vi "Begin.vi"(8 "error in":errorcluster) -> (0 "error out":errorcluster)   [LabVIEW 2014]
doc: "Called before other user functions, this VI is expected to open initial I/O refnums, load in file data, and do all program initialization. Notice that the <B>error out</B> terminal is simply used for data flow. Wiring it to other structures or subVIs ensures that this VI runs first."
uses:
  <vilib>/Rock Robotics/WPI/DriverStation/WPI_DriverStationRobotMode2.ctl
  <vilib>/Rock Robotics/WPI/Joystick/WPI_JoystickDeviceEnum.ctl
  <vilib>/Rock Robotics/SystemInterfaces/DIO/FPGA_DIOChannel.ctl
  <vilib>/Rock Robotics/SystemInterfaces/Typedef/FPGA_TypedefDigitalModule.ctl
  <vilib>/Rock Robotics/WPI/SafetyOutput/WPI_SafetyOutputConfigMenu.ctl
  <vilib>/Rock Robotics/SystemInterfaces/DIO/FPGA_DIOPWMChannel.ctl
  <vilib>/Rock Robotics/WPI/Solenoid/WPI_SolenoidChannel.ctl
  Robot Global Data.vi
  <vilib>/Rock Robotics/Network Tables/SD Write String Array.vi
  <vilib>/Rock Robotics/WPI/RobotDrive/WPI_RobotDriveOpen4MotorWithCANTalonSRX.vi
  <vilib>/Rock Robotics/WPI/RobotDrive/WPI_RobotDriveOpen2MotorWithCANTalonSRX.vi
  <vilib>/Rock Robotics/WPI/Switch/WPI_SwitchOpenLimit.vi
  <vilib>/Rock Robotics/WPI/Solenoid/WPI_SolenoidOpenDouble.vi
  <vilib>/Rock Robotics/WPI/Compressor/WPI_CompressorGetSetRefNum.vi
  <vilib>/Rock Robotics/WPI/MotorControl/WPI_MotorControlOpen VictorSP.vi
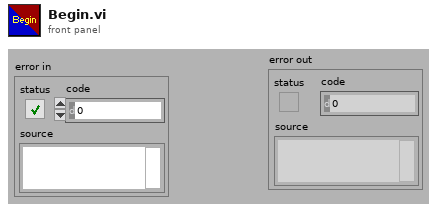
[diagram p1: front panel]
types:
  T1 = typedef "WPI_SolenoidChannel.ctl" = enum8{"Solenoid 0", "Solenoid 1", "Solenoid 2", "Solenoid 3", "Solenoid 4", "Solenoid 5", "Solenoid 6", "Solenoid 7", "Invalid"}
  T2 = typedef "FPGA_DIOChannel.ctl" = enum8{"DIO 0", "DIO 1", "DIO 2", "DIO 3", "DIO 4", "DIO 5", "DIO 6", "DIO 7", "DIO 8", "DIO 9", "DIO MXP 0", "DIO MXP 1", "DIO MXP 2", "DIO MXP 3", "DIO MXP 4", "DIO MXP 5", "DIO MXP 6", "DIO MXP 7", "DIO MXP 8", "DIO MXP 9", "DIO MXP 10", "DIO MXP 11", "DIO MXP 12", "DIO MXP 13", "DIO MXP 14", "DIO MXP 15", "Invalid"}
  T3 = typedef "FPGA_TypedefDigitalModule.ctl" = enum16{"Controller 1"}
  T4 = typedef "FPGA_DIOPWMChannel.ctl" = enum8{"PWM 0", "PWM 1", "PWM 2", "PWM 3", "PWM 4", "PWM 5", "PWM 6", "PWM 7", "PWM 8", "PWM 9", "PWM MXP 0", "PWM MXP 1", "PWM MXP 2", "PWM MXP 3", "PWM MXP 4", "PWM MXP 5", "PWM MXP 6", "PWM MXP 7", "PWM MXP 8", "PWM MXP 9", "Invalid"}
  T5 = typedef "WPI_SafetyOutputConfigMenu.ctl" = enum16{"Enable", "Disable"}
  T6 = typedef "WPI_JoystickDeviceEnum.ctl" = enum16{"USB 0", "USB 1", "USB 2", "USB 3", "USB 4", "USB 5"}
  T7 = typedef "WPI_DriverStationRobotMode2.ctl" = enum16{"Autonomous Disabled", "Autonomous Enabled", "Teleop Disabled", "Teleop Enabled", "Disconnected", "Finish", "Test Disabled", "Test Enabled", "Emergency Stopped"}
  T8 = typedef "WPI_MotorControlDeviceRef.ctl" = cluster{"DeviceStatus":errorcluster, "Type":T9, "PWM":cluster{"Controller":T3, "PWM Channel":T4, "DeadBand":T10}, "CAN":cluster{"Device Number":u8, "Control Mode":T11, "Semaphore":T12, "Max Vout":dbl, "TalonSRX Control Mode":T13}, "Invert":bool, "TransformRef":T14, "InvTransformRef":T14}
  T9 = typedef "WPI_MotorControlType.ctl" = enum16{"PWM", "CAN", "CANTalonSRX"}
  T10 = typedef "WPI_PWMDeadband.ctl" = cluster{"Name":string, "maxPositivePwm":i32, "minPositivePwm":i32, "centerPwm":i32, "maxNegativePwm":i32, "minNegativePwm":i32, "angularRange":u16}
  T11 = typedef "WPI_CANJaguar_ControlMode.ctl" = enum8{"Percent VBus", "Current", "Speed", "Position", "Voltage"}
  T12 = typedef "Semaphore RefNum" = refnum<k1>
  T13 = typedef "WPI_CANTalonSRX_APIControlMode.ctl" = enum8{"Percent VBus", "Speed", "Position", "Slave", "Unchanged / Invalid"}
  T14 = typedef "WPI_PWMTransform_ConPane.ctl" = refnum<vi>
  T15 = typedef "WPI_RobotDriveDevRef.ctl" = cluster{"DevStatus":errorcluster, "Motors[]":T8[], "Square Inputs":bool, "Max Output":dbl}
  T16 = typedef "WPI_CompressorDevRef.ctl" = cluster{"DevStatus":errorcluster, "Pneumatics Control Module":u8}
  T17 = typedef "WPI_ServoDeviceRef.ctl" = cluster{"DeviceStatus":errorcluster, "Controller":T3, "PWM Channel":T4, "DeadBand":T10}
  T18 = typedef "WPI_JoystickDevRef.ctl" = cluster{"Device":T6}
  T19 = typedef "WPI_DigitalInputDevRef.ctl" = cluster{"DevStatus":errorcluster, "DIO Channel":T2, "Controller":T3}
  T20 = typedef "WPI_SolenoidDevRef.ctl" = cluster{"DevStatus":errorcluster, "Pneumatics Control Module":u8, "Forward Solenoid Channel":T1, "Reverse Solenoid Channel":T1}
  T21 = typedef "WPI_SwitchDevRef.ctl" = cluster{"DevStatus":errorcluster, "DIO Channel":T2, "Controller":T3, "CntIndex":T22, "Normally Closed":bool}
  T22 = typedef "FPGA_CounterCtrSystemIndex.ctl" = enum8{"Ctr 0", "Ctr 1", "Ctr 2", "Ctr 3", "Ctr 4", "Ctr 5", "Ctr 6", "Ctr 7", "Invalid"}
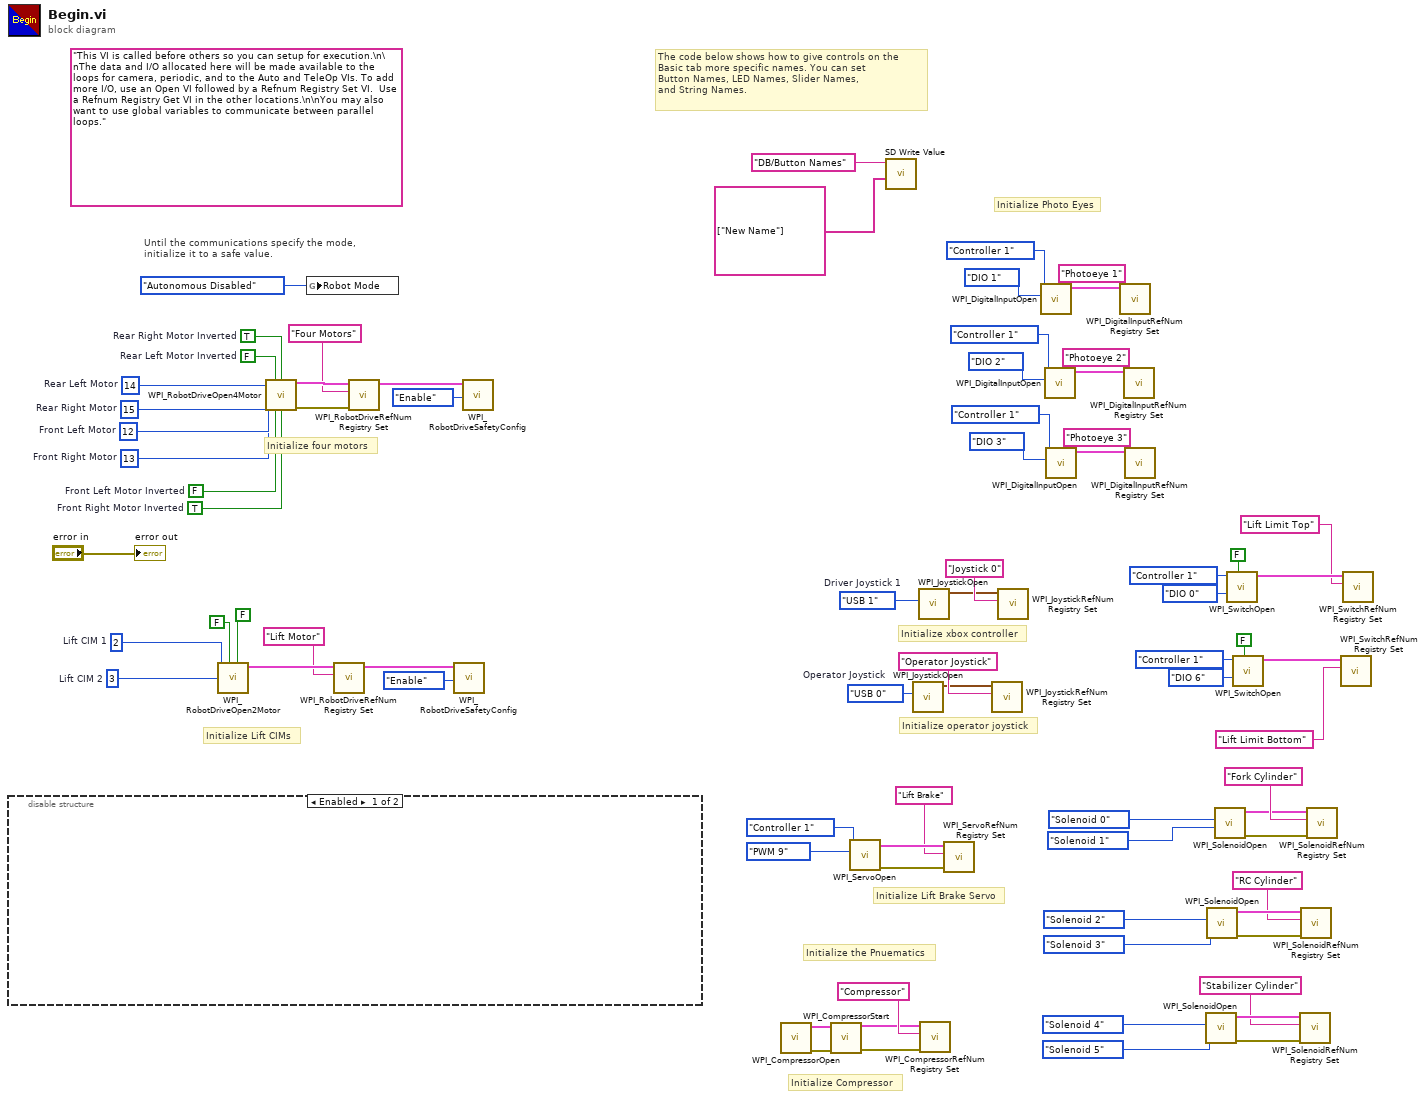
[diagram p0: block diagram]
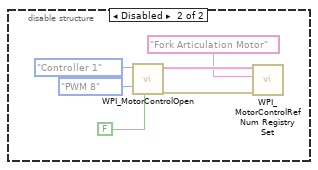
[diagram p2: hidden frame]
diagram:
  w38 = u8 3  # Lift CIM 2
  w37 = u8 2  # Lift CIM 1
  w56 = u8 13  # Front Right Motor
  w57 = u8 12  # Front Left Motor
  w58 = u8 15  # Rear Right Motor
  w59 = u8 14  # Rear Left Motor
  w60 = WPI_JoystickDeviceEnum."USB 0"  # Operator Joystick
  w63 = TRUE  # Front Right Motor Inverted
  w64 = FALSE  # Front Left Motor Inverted
  w65 = TRUE  # Rear Right Motor Inverted
  w66 = FALSE  # Rear Left Motor Inverted
  w70 = WPI_JoystickDeviceEnum."USB 1"  # Driver Joystick 1
  (unwired) "This VI is called before others so you can setup for execution.\n\nThe data and I/O allocated here will be made available to the loops for camera, periodic, and to the Auto and TeleOp VIs. To add more I/O, use an Open VI followed by a Refnum Registry Set VI.  Use a Refnum Registry Get VI in the other locations.\n\nYou may also want to use global variables to communicate between parallel loops."
  # "Initialize Compressor"
  # "Initialize the Pnuematics"
  # "Initialize Photo Eyes"
  # "Initialize Lift Brake Servo"
  # "Initialize Lift CIMs"
  # "Initialize operator joystick"
  # "The code below shows how to give controls on the\nBasic tab more specific names. You can set\nButton Names, LED Names, Slider Names,\nand String Names."
  # "Initialize xbox controller"
  # "Until the communications specify the mode,\ninitialize it to a safe value."
  # "Initialize four motors"
  n1 = disable-structure shown="Enabled" {
    frame Enabled {
    }
    frame Disabled {
      n2 = call-poly <vilib>:"WPI_MotorControlOpen.vi"("Invert"=FALSE, "PWM Channel"=FPGA_DIOPWMChannel."PWM 8", "Controller"=FPGA_TypedefDigitalModule."Controller 1") -> ("error out"=w79:errorcluster, "MotorControlDeviceRef"=w82:T8)  [unwired: 7 in]
      n3 = call <vilib>:"WPI_MotorControlRefNum Registry Set.vi"("error in (no error)"=w79, "refnum name"="Fork Articulation Motor", "MotorControlDevRef"=w82) -> ()  [unwired: 7 in, 2 out]
    }
  }
  n4 = call-poly <vilib>:"WPI_RobotDriveOpen2Motor.vi"("Right Motor Inverted"=FALSE, "Left Motor Inverted"=FALSE, "Right Motor"=w38, "Left Motor"=w37) -> ("RobotDriveDevRef"=w41:T15)  [unwired: 6 in, 1 out]
  n5 = call-poly <vilib>:"WPI_RobotDriveOpen4Motor.vi"("Rear Left Motor"=w59, "Rear Left Motor Inverted"=w66, "Rear Right Motor Inverted"=w65, "Rear Right Motor"=w58, "Front Left Motor"=w57, "Front Right Motor"=w56, "Front Left Motor Inverted"=w64, "Front Right Motor Inverted"=w63) -> ("RobotDriveDevRef"=w78:T15, "error out"=w76:errorcluster)  [unwired: 6 in]
  n6 = global write "Robot Global Data.vi" "Robot Mode"(WPI_DriverStationRobotMode2."Autonomous Disabled" ("Robot Mode")) -> ()
  n7 = call <vilib>:"WPI_RobotDriveRefNum Registry Set.vi"("refnum name"="Lift Motor", "RobotDriveDevRef"=w41) -> ("RobotDriveDevRef"=w43:T15)  [unwired: 8 in, 1 out]
  n8 = call <vilib>:"WPI_RobotDriveRefNum Registry Set.vi"("error in (no error)"=w76, "refnum name"="Four Motors", "RobotDriveDevRef"=w78) -> ("RobotDriveDevRef"=w75:T15)  [unwired: 8 out]
  n9 = call <vilib>:"WPI_RobotDriveSafetyConfig.vi"("mode"=WPI_SafetyOutputConfigMenu."Enable", "RobotDriveDevRef"=w43) -> ()  [unwired: 8 in, 2 out]
  n10 = call <vilib>:"WPI_RobotDriveSafetyConfig.vi"("mode"=WPI_SafetyOutputConfigMenu."Enable", "RobotDriveDevRef"=w75) -> ()  [unwired: 8 in, 2 out]
  n11 = call <vilib>:"WPI_CompressorOpen.vi"() -> ("CompressorDevRef"=w18:T16, "error out"=w11:errorcluster)  [unwired: 14 in]
  n12 = call <vilib>:"WPI_CompressorStart.vi"("error in (no error)"=w11, "CompressorDevRef"=w18) -> ("error out"=w12:errorcluster, "CompressorDevRef"=w13:T16)  [unwired: 8 out]
  n13 = call <vilib>:"WPI_ServoOpen.vi"("PWM Channel"=FPGA_DIOPWMChannel."PWM 9", "Controller"=FPGA_TypedefDigitalModule."Controller 1") -> ("error out"=w21:errorcluster, "ServoDeviceRef"=w33:T17)  [unwired: 8 in]
  n14 = call-poly <vilib>:"SD Write Value.vi"("String Array"=string[] ["New Name"], "Name"="DB/Button Names") -> ()  [unwired: 8 in, 2 out]
  n15 = call <vilib>:"WPI_JoystickOpen.vi"("JoystickDevice"=w60) -> ("JoystickDevRef"=w61:T18)  [unwired: 10 in]
  n16 = call <vilib>:"WPI_JoystickOpen.vi"("JoystickDevice"=w70) -> ("JoystickDevRef"=w71:T18)  [unwired: 10 in]
  n17 = call <vilib>:"WPI_CompressorRefNum Registry Set.vi"("error in (no error)"=w12, "refnum name"="Compressor", "CompressorDevRef"=w13) -> ()  [unwired: 7 in, 2 out]
  n18 = call <vilib>:"WPI_ServoRefNum Registry Set.vi"("error in (no error)"=w21, "refnum name"="Lift Brake", "ServoDeviceRef"=w33) -> ()  [unwired: 7 in, 2 out]
  n19 = call <vilib>:"WPI_JoystickRefNum Registry Set.vi"("refnum name"="Operator Joystick", "JoystickDevRef"=w61) -> ()  [unwired: 8 in, 2 out]
  n20 = call <vilib>:"WPI_JoystickRefNum Registry Set.vi"("refnum name"="Joystick 0", "JoystickDevRef"=w71) -> ()  [unwired: 8 in, 2 out]
  n21 = call <vilib>:"WPI_DigitalInputOpen.vi"("DIO Channel"=FPGA_DIOChannel."DIO 1", "Controller"=FPGA_TypedefDigitalModule."Controller 1") -> ("DigitalInputDevRef"=w47:T19)  [unwired: 8 in, 1 out]
  n22 = call <vilib>:"WPI_DigitalInputOpen.vi"("DIO Channel"=FPGA_DIOChannel."DIO 2", "Controller"=FPGA_TypedefDigitalModule."Controller 1") -> ("DigitalInputDevRef"=w55:T19)  [unwired: 8 in, 1 out]
  n23 = call <vilib>:"WPI_DigitalInputOpen.vi"("DIO Channel"=FPGA_DIOChannel."DIO 3", "Controller"=FPGA_TypedefDigitalModule."Controller 1") -> ("DigitalInputDevRef"=w51:T19)  [unwired: 8 in, 1 out]
  n24 = call <vilib>:"WPI_DigitalInputRefNum Registry Set.vi"("refnum name"="Photoeye 1", "DigitalInputDevRef"=w47) -> ()  [unwired: 8 in, 2 out]
  n25 = call <vilib>:"WPI_DigitalInputRefNum Registry Set.vi"("refnum name"="Photoeye 2", "DigitalInputDevRef"=w55) -> ()  [unwired: 8 in, 2 out]
  n26 = call <vilib>:"WPI_DigitalInputRefNum Registry Set.vi"("refnum name"="Photoeye 3", "DigitalInputDevRef"=w51) -> ()  [unwired: 8 in, 2 out]
  n27 = call-poly <vilib>:"WPI_SolenoidOpen.vi"("Reverse Solenoid Channel"=WPI_SolenoidChannel."Solenoid 5", "Forward Solenoid Channel"=WPI_SolenoidChannel."Solenoid 4" ("Solenoid Channel")) -> ("error out"=w4:errorcluster, "SolenoidDevRef"=w5:T20)  [unwired: 2 in, 6 out]
  n28 = call-poly <vilib>:"WPI_SolenoidOpen.vi"("Reverse Solenoid Channel"=WPI_SolenoidChannel."Solenoid 3", "Forward Solenoid Channel"=WPI_SolenoidChannel."Solenoid 2" ("Solenoid Channel")) -> ("error out"=w9:errorcluster, "SolenoidDevRef"=w10:T20)  [unwired: 2 in, 6 out]
  n29 = call-poly <vilib>:"WPI_SolenoidOpen.vi"("Reverse Solenoid Channel"=WPI_SolenoidChannel."Solenoid 1" ("Extend Solenoid Channel"), "Forward Solenoid Channel"=WPI_SolenoidChannel."Solenoid 0" ("Retract Solenoid Channel")) -> ("error out"=w15:errorcluster, "SolenoidDevRef"=w16:T20)  [unwired: 2 in, 6 out]
  n30 = call-poly <vilib>:"WPI_SwitchOpen.vi"("Normally Closed"=FALSE, "DIO Channel"=FPGA_DIOChannel."DIO 0", "Controller"=FPGA_TypedefDigitalModule."Controller 1") -> ("SwitchDevRef"=w24:T21)  [unwired: 7 in, 1 out]
  n31 = call-poly <vilib>:"WPI_SwitchOpen.vi"("Normally Closed"=FALSE, "DIO Channel"=FPGA_DIOChannel."DIO 6", "Controller"=FPGA_TypedefDigitalModule."Controller 1") -> ("SwitchDevRef"=w25:T21)  [unwired: 7 in, 1 out]
  n32 = call <vilib>:"WPI_SolenoidRefNum Registry Set.vi"("error in (no error)"=w4, "refnum name"="Stabilizer Cylinder", "SolenoidDevRef"=w5) -> ()  [unwired: 7 in, 2 out]
  n33 = call <vilib>:"WPI_SolenoidRefNum Registry Set.vi"("error in (no error)"=w9, "refnum name"="RC Cylinder", "SolenoidDevRef"=w10) -> ()  [unwired: 7 in, 2 out]
  n34 = call <vilib>:"WPI_SolenoidRefNum Registry Set.vi"("error in (no error)"=w15, "refnum name"="Fork Cylinder", "SolenoidDevRef"=w16) -> ()  [unwired: 7 in, 2 out]
  n35 = call <vilib>:"WPI_SwitchRefNum Registry Set.vi"("refnum name"="Lift Limit Bottom", "SwitchDevRef"=w25) -> ()  [unwired: 8 in, 2 out]
  n36 = call <vilib>:"WPI_SwitchRefNum Registry Set.vi"("refnum name"="Lift Limit Top", "SwitchDevRef"=w24) -> ()  [unwired: 8 in, 2 out]
  "error out" <- "error in"
